vi "StatusRegisterSet.vi"(8 "错误输入（无错误）":errorcluster, 10 "设置寄存器使能值命令":string, 11 "VISA引用句柄输入":refnum<visa-resource-name>) -> (0 "错误输出":errorcluster, 3 "VISA引用句柄输出":refnum<visa-resource-name>)   [LabVIEW 2018]
doc: "设置事件状态寄存器和状态寄存器的使能值"
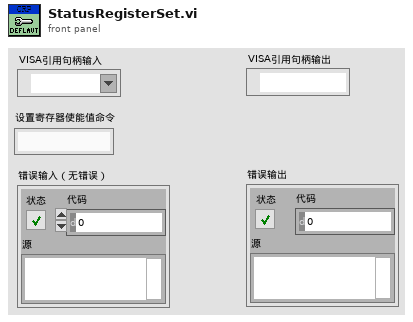
[diagram p1: front panel]
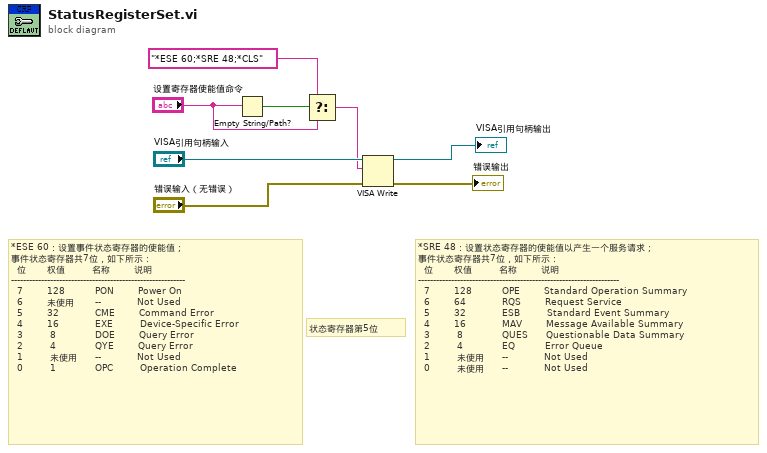
[diagram p0: block diagram]
diagram:
  # "状态寄存器第5位"
  # "*SRE 48：设置状态寄存器的使能值以产生一个服务请求；\n事件状态寄存器共7位，如下所示： \n  位       权值         名称        说明\n-------------------------------------------------------------------\n  7        128          OPE        Standard Operation Summary  \n  6        64            RQS        Request Service       \n  5        32            ESB         Standard Event Summary\n  4        16            MAV        Message Available Summary\n  3         8             QUES      Questionable Data Summary\n  2         4             EQ          Error Queue\n  1         未使用      --            Not Used\n  0         未使用      --            Not Used"
  # "*ESE 60：设置事件状态寄存器的使能值；\n事件状态寄存器共7位，如下所示： \n  位       权值         名称        说明\n----------------------------------------------------------\n  7        128          PON        Power On  \n  6        未使用       --            Not Used\n  5        32            CME        Command Error\n  4        16            EXE         Device-Specific Error\n  3         8             DOE        Query Error\n  2         4             QYE        Query Error\n  1         未使用      --            Not Used\n  0         1             OPC         Operation Complete"
  n1 = Empty String/Path?(string/path="设置寄存器使能值命令") -> (empty?=w3:bool)
  n2 = Select(t="*ESE 60;*SRE 48;*CLS" ("SCPI字符串"), s=w3, f="设置寄存器使能值命令") -> (s? t:f=w4:string)
  n3 = VISA Write(VISA resource name="VISA引用句柄输入", write buffer=w4, error in (no error)="错误输入（无错误）") -> (VISA resource name out=→"VISA引用句柄输出":refnum<visa-resource-name>, error out=→"错误输出":errorcluster)  [unwired: 1 out]
